vi "Create Data Channel - Single Channel - Comparison.vi"(8 "error in (no error)":errorcluster, 9 "settings":T2, 10 "channel name":string, 11 "response refnum in":T1 format="%.0x") -> (0 "error out":errorcluster, 2 "channel refnum":T1 format="%.0x", 3 "response refnum out":T1 format="%.0x")   [LabVIEW 2018, in "Instrument Addon Scripting API.lvlib"]
doc: "Creates a new Data Channel with the following configuration: \nData Type: Single Channel\nChannel Type: Comparison\n\nInput: \nMessage Refnum In: reference to the \"Response\" message.\nName: represents the desired name of the channel.\nSettings: represents the settings applied on the new channel.\n\nOutput:\nMessage Refnum Out: reference to the \"Response\" message used as input.\nChannel Refnum: reference to the newly created channel."
uses:
  Instrument Addon Scripting API.lvlib
  TypeDefs/Single Channel Comparison Settings.ctl
  <vilib>/NI Veristand/Custom Device API/Custom Device Item Ref.ctl
  Addon/Addon Shared/Types/Data Parameters.ctl
  Addon/Addon Shared/Types/Protocol Data Type.ctl
  Addon/Addon Shared/Types/Data Channel Type.ctl
  Addon/Addon Shared/Types/Type Cast Type.ctl
  Addon/Addon Shared/Types/Endian.ctl
  <vilib>/NI Veristand/Custom Device API/Custom Device Channel.ctl
  <vilib>/NI Veristand/Custom Device API/Custom Device Channel Type.ctl
  <vilib>/NI Veristand/Custom Device API/Custom Device API.lvlib
  Addon/Addon Shared/Instrument Addon Shared.lvlib
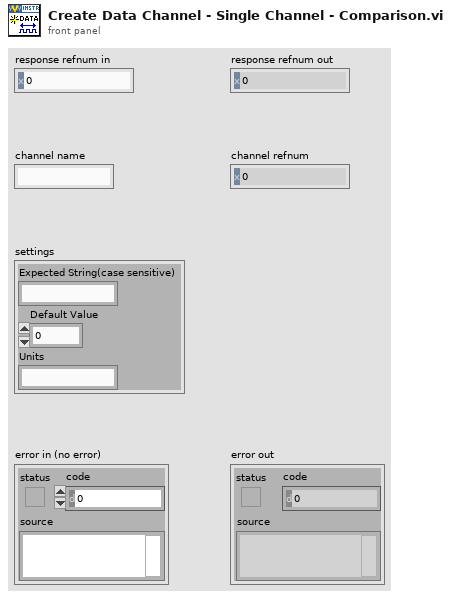
[diagram p1: front panel]
types:
  T1 = typedef "Custom Device API.lvlib/Custom Device Item Ref.ctl" = u64
  T2 = typedef "Instrument Addon Scripting API.lvlib/Single Channel Comparison Settings.ctl" = cluster{"Expected String(case sensitive)":string, "Default Value":dbl, "Units":string}
  T3 = typedef "Instrument Addon Shared.lvlib/Data Channel Type.ctl" = enum16{"Format", "Comparison", "Type Cast", "Enumerated List"}
  T4 = typedef "Instrument Addon Shared.lvlib/Protocol Data Type.ctl" = enum16{"Single Channel", "Array"}
  T5 = typedef "Custom Device API.lvlib/Custom Device Channel.ctl" = cluster{"Type":T6, "Units":string, "Default Value":dbl, "Faultable":bool, "Scalable":bool}
  T6 = typedef "Custom Device API.lvlib/Custom Device Channel Type.ctl" = enum16{"Input", "Output"}
  T7 = typedef "Instrument Addon Shared.lvlib/Data Parameters.ctl" = cluster{"Data Type":T4, "Channel Type":T3, "Format String":string, "Expected String":string, "Type":T8, "List":string[], "Delimiter":string, "Endian":T9}
  T8 = typedef "Instrument Addon Shared.lvlib/Type Cast Type.ctl" = enum16{"DBL", "SGL", "U64", "U32", "U16", "U8", "I64", "I32", "I16", "I8"}
  T9 = typedef "Instrument Addon Shared.lvlib/Endian.ctl" = enum16{"Native", "Little", "Big"}
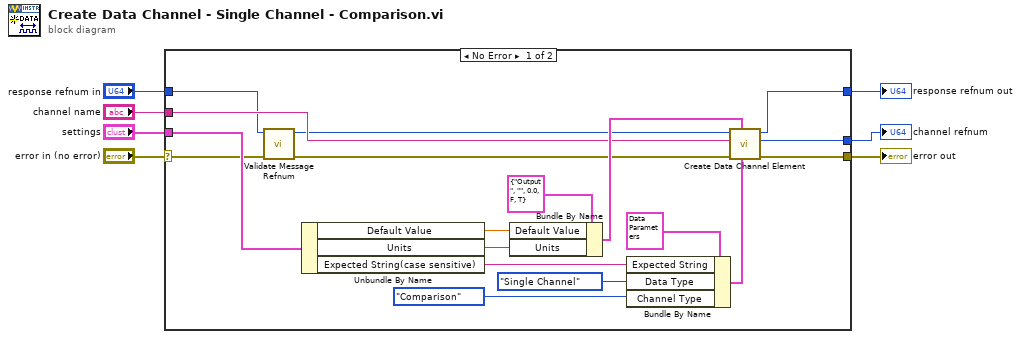
[diagram p0: block diagram]
diagram:
  n1 = case shown="No Error" "error in (no error)" {
    selector: "error in (no error)" -> [w12 w26]
    tunnel: [w16 w26] -> w7
    tunnel: "settings" -> [w23 _]
    tunnel: [w14 w27] -> w5
    tunnel: [w13 _] -> w4
    tunnel: "channel name" -> [w10 _]
    tunnel: "response refnum in" -> [w8 w27]
    frame No Error {
      n2 = call "Validate Message Refnum.vi"("error in (no error)"=w12, "Message in"=w8) -> ("error out"=w11:errorcluster, "Message out"=w9:T1)  [unwired: 8 in]
      n3 = Unbundle By Name(w23) -> ("Default Value"=w22:dbl, "Units"=w21:string, "Expected String(case sensitive)"=w20:string)
      n4 = Bundle By Name(cluster=T5 {"Type"=enum."Output", "Units"="", "Default Value"=0.0, "Faultable"=FALSE, "Scalable"=TRUE} ("Channel"), "Default Value"=w22, "Units"=w21) -> (w17:T5)
      n5 = Bundle By Name(cluster=T7 {"Data Type"=enum."Single Channel", "Channel Type"=enum."Format", "Format String"="%.3g", "Expected String"="", "Type"=enum."SGL", "List"=[], "Delimiter"=",", "Endian"=enum."Native"} ("Data Parameters"), "Expected String"=w20, "Data Type"=Protocol_Data_Type."Single Channel", "Channel Type"=Data_Channel_Type."Comparison") -> (w15:T7)
      n6 = call "Create Data Channel Element.vi"("Data Channel Parameters"=w15, "Settings"=w17, "Error In"=w11, "Name"=w10, "Refnum In"=w9) -> ("Error Out"=w16:errorcluster, "Channel Refnum"=w13:T1, "Refnum Out"=w14:T1)  [unwired: 4 in]
    }
    frame Error {
    }
  }
  "error out" <- w7
  "response refnum out" <- w5
  "channel refnum" <- w4
